vi "Refresh User.vi"(8 "error in (no error)":errorcluster, 10 "User In":refnum<class "User.lvclass">, 11 "InMemoryUserProvider in":refnum<class "InMemoryUserProvider.lvclass">) -> (0 "error out":errorcluster, 2 "User":refnum<class "User.lvclass">, 3 "InMemoryUserProvider out":refnum<class "InMemoryUserProvider.lvclass">)   [LabVIEW 2020, in "HTTP Server.lvlib" / "InMemoryUserProvider.lvclass"]
uses:
  InMemoryUserProvider.lvclass
  User/User.lvclass
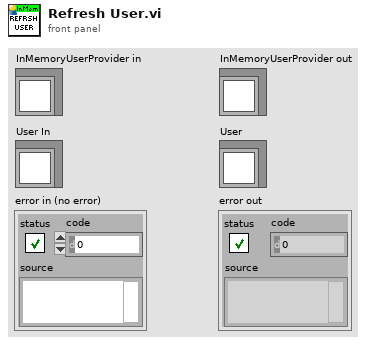
[diagram p1: front panel]
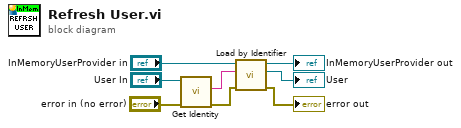
[diagram p0: block diagram]
diagram:
  n1 = call-dynamic "Get Identity.vi"("error in (no error)"="error in (no error)", "User in"="User In") -> ("error out"=w3:errorcluster, "Identity"=w6:string)  [unwired: 7 in, 1 out]
  n2 = call-dynamic "Load by Identifier.vi"("error in (no error)"=w3, "Identifier"=w6, "InMemoryUserProvider in"="InMemoryUserProvider in") -> ("error out"=→"error out":errorcluster, "User"=→"User":refnum<class "User.lvclass">, "InMemoryUserProvider out"=→"InMemoryUserProvider out":refnum<class "InMemoryUserProvider.lvclass">)  [unwired: 6 in]
